vi "get runtime class name.vi"(8 "error in":errorcluster, 11 "configuration in":refnum<class "PL_System Configuration.lvclass">) -> (0 "error out":errorcluster, 2 "class name":string, 3 "configuration out":refnum<class "PL_System Configuration.lvclass">)   [LabVIEW 2013, in "PL_System Configuration.lvclass"]
doc: "Provides an interface for determining the runtime class associated with this configuration. This class name can then be used to dynamically load or locate the runtime class for initialization purposes."
uses:
  PL_System Configuration.lvclass
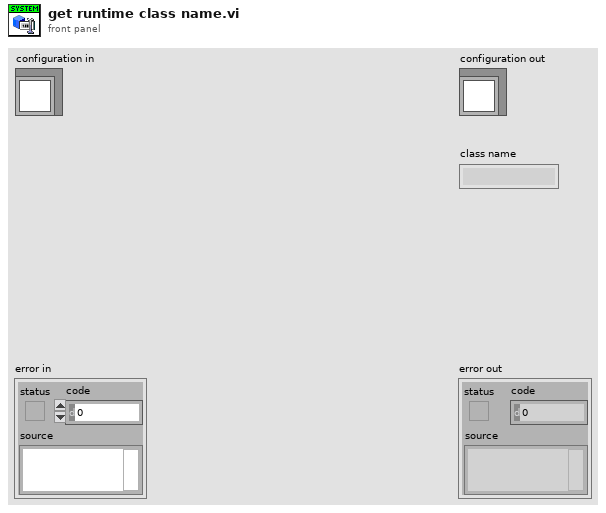
[diagram p1: front panel]
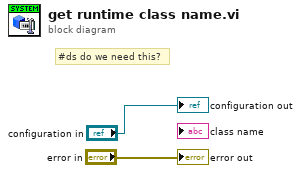
[diagram p0: block diagram]
diagram:
  # "#ds do we need this?"
  "error out" <- "error in"
  "configuration out" <- "configuration in"
